vi "Load.vi"(7 "Wait For Load (T)":bool=TRUE, 8 "error in (no error)":errorcluster, 10 "Path":string, 11 "Channel in":refnum<data-value>) -> (0 "error out":errorcluster, 3 "Channel out":refnum<data-value>)   [LabVIEW 2020, in "G-Audio.lvlib" / "Channel.lvclass"]
uses:
  Channel.lvclass
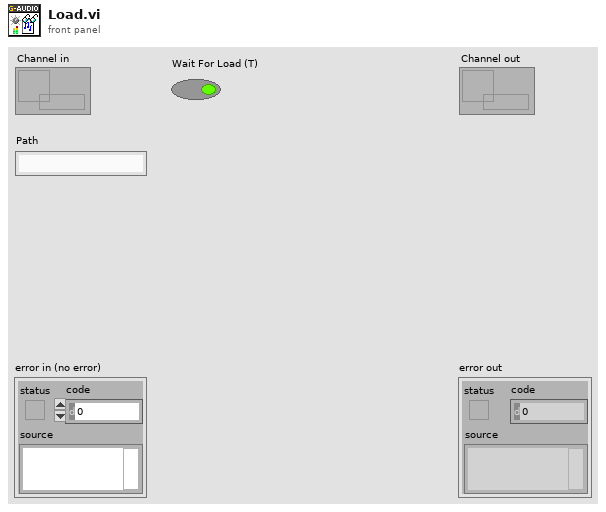
[diagram p1: front panel]
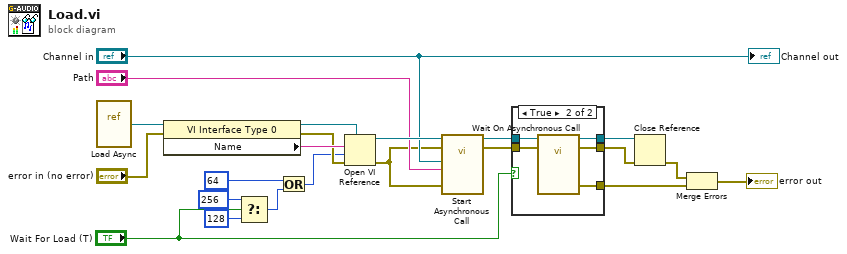
[diagram p0: block diagram]
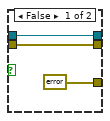
[diagram p2: hidden frame]
diagram:
  n1 = vi-ref "Load Async.vi"() -> (w22:refnum<vi>)
  n2 = property class="VI Interface Type 0"(reference=w22, error in="error in (no error)") -> (reference out=w20:refnum<vi>, error out=w18:errorcluster, "Name"=w21:string)
  n3 = Select(t=256 ("options"), s="Wait For Load (T)", f=128 ("options")) -> (s? t:f=w8:i32)
  n4 = Or(x=64 ("options"), y=w8) -> (x .or. y?=w14:i32)
  n5 = Open VI Reference(type specifier VI Refnum (for type only)=w20, vi path=w21, options=w14, error in (no error)=w18) -> (vi reference=w19:refnum<vi>, error out=w1:errorcluster)  [unwired: 2 in]
  n6 = call-by-ref "Start Asynchronous Call"(reference=w19, error in=w1, 8:"error in (no error)"=w1, "String"="Path", "Channel in"="Channel in") -> (reference out=w11:refnum<vi>, error out=w12:errorcluster)  [unwired: 7 in, 2 out]
  n7 = case shown="True" "Wait For Load (T)" {
    tunnel: w12 -> [w25 w30]
    tunnel: w11 -> [w24 w29]
    tunnel: [w25 w28] -> w5
    tunnel: [w24 w27] -> w6
    tunnel: [errorcluster {"status"=FALSE, "code"=0, "source"=""} ("error out") w26] -> w4
    frame False {
    }
    frame True {
      n8 = call-by-ref "Wait On Asynchronous Call"(reference=w29, error in=w30) -> (reference out=w27:refnum<vi>, error out=w28:errorcluster, 0:"error out"=w26:errorcluster)  [unwired: 10 in, 1 out]
    }
  }
  n9 = Close Reference(reference=w6, error in (no error)=w5) -> (error out=w3:errorcluster)
  n10 = Merge Errors(w3, w4) -> (→"error out":errorcluster)
  "Channel out" <- "Channel in"
